vi "Read Page Info.vi"(7 "IFDOffset":u32, 8 "error in (no error)":errorcluster, 9 "Tiff Bitness":T1(ring), 11 "Byte Stream File in":refnum<file>) -> (0 "error in (no error) 2":errorcluster, 1 "Page Info":T3(array[cluster]), 2 "N Pages":i32, 3 "Byte Stream File out":refnum<file>)   [LabVIEW 2020, in "LV Tiff.lvlib"]
uses:
  LV Tiff.lvlib
  Tiff Data Type.ctl
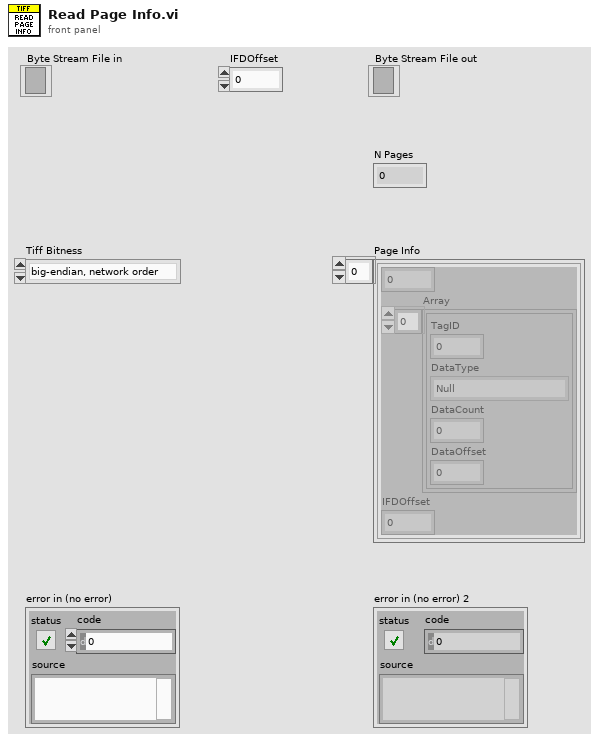
[diagram p1: front panel]
types:
  T1 = enum16{"big-endian, network order", "native, host order", "little-endian"}
  T2 = typedef "LV Tiff.lvlib/Tiff Data Type.ctl" = enum16{"Null", "BYTE", "ASCII", "SHORT", "LONG", "RATIONAL", "SBYTE", "UNDEFINE", "SSHORT", "SLONG", "SRATIONAL", "FLOAT", "DOUBLE"}
  T3 = cluster{i32, "Array":cluster{"TagID":u16, "DataType":T2, "DataCount":u32, "DataOffset":u32}[], "IFDOffset":u32}[]
  T4 = cluster{"TagID":u16, "DataType":T2, "DataCount":u32, "DataOffset":u32}[]
  T5 = cluster{i32, "Array":cluster{"TagID":u16, "DataType":T2, "DataCount":u32, "DataOffset":u32}[], "IFDOffset":u32}
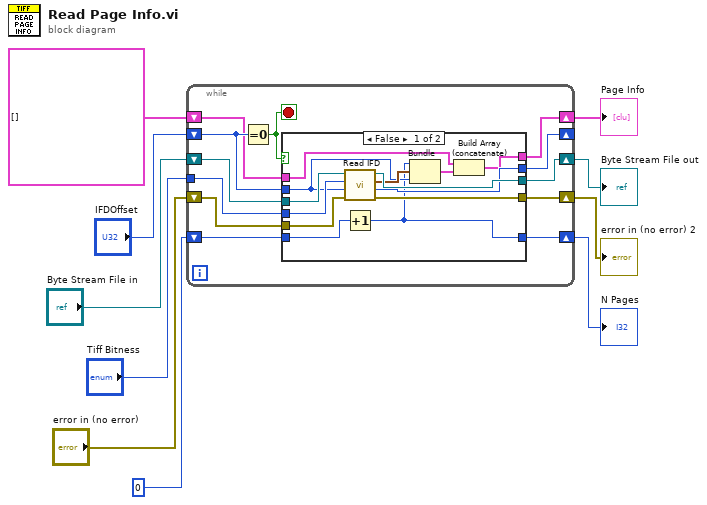
[diagram p0: block diagram]
diagram:
  n1 = while {
    tunnel: "Tiff Bitness" -> [w21]
    shift-right: [w20] -> _
    shift-left: "IFDOffset" -> [w19]
    shift-right: [w18] -> w8
    shift-left: "Byte Stream File in" -> [w22]
    shift-right: [w16] -> w1
    shift-left: "error in (no error)" -> [w17]
    shift-right: [w14] -> w6
    shift-left: 0 ("Numeric in") -> [w13]
    shift-right: [w12] -> w10
    shift-left: T3 [] -> [w11]
    stop <- w15 stop-if-true
    n2 = Equal To 0?(x=w19) -> (x = 0?=w15:bool)
    n3 = case shown="False" w15 {
      tunnel: w22 -> [w35 w38]
      tunnel: w21 -> [w34 _]
      tunnel: [w28 w39] -> w20
      tunnel: w19 -> [w27 w39]
      tunnel: [w33 w38] -> w18
      tunnel: w17 -> [w32 w40]
      tunnel: [w31 w40] -> w16
      tunnel: [w26 w37] -> w14
      tunnel: w13 -> [w30 w37]
      tunnel: [w24 w36] -> w12
      tunnel: w11 -> [w23 w36]
      frame False {
        n4 = call "Read IFD.vi"("error in"=w32, "IFDOffset"=w27, "Tiff Bitness"=w34, "Byte Stream File in"=w35) -> ("error out"=w31:errorcluster, "NextIDOOffset"=w28:u32, "Array"=w29:T4, "refnum out"=w33:refnum<file>)  [unwired: 4 in]
        n5 = Increment(x=w30) -> (x+1=w26:i32)
        n6 = Bundle(w26, "Array"=w29, "IFDOffset"=w27) -> (w25:T5)  [unwired: 1 in]
        n7 = Build Array (concatenate)(w23, w25) -> (w24:T3)
      }
      frame True {
      }
    }
  }
  "Page Info" <- w10
  "Byte Stream File out" <- w8
  "N Pages" <- w6
  "error in (no error) 2" <- w1
